vi "IMAQ-SaveVideo.vi"(1 "Exposure Time (ms)":u32, 2 "Image":T1, 3 "Grabar":refnum<vi>, 4 "Compression Filter":string) -> (0 "Selected Path for AVI":path)   [LabVIEW 2010]
uses:
  <vilib>/vision/Image Controls.llb/IMAQ Image.ctl
  <vilib>/vision/Avi1.llb/AviRefnum.ctl
  <vilib>/Utility/error.llb/DialogType.ctl
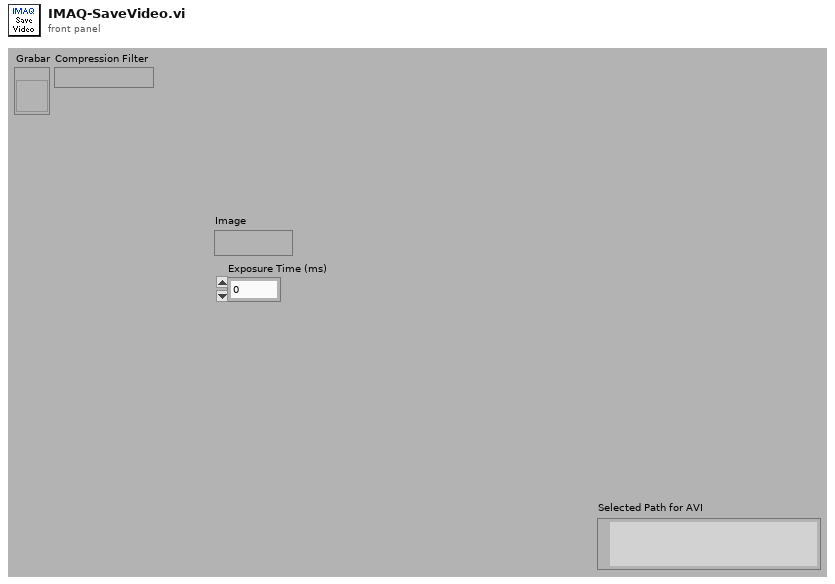
[diagram p1: front panel]
types:
  T1 = typedef "IMAQ Image.ctl" = refnum<image>
  T2 = typedef "AviRefnum.ctl" = refnum<k1>
  T3 = enum32{"existing file", "new file", "new or existing file", "existing dir", "new dir", "new or existing dir", "existing file (use LLBs)", "new file (use LLBs)", "new or existing file (use LLBs)", "new or existing file or directory (use LLBs)"}
  T4 = typedef "DialogType.ctl" = u16
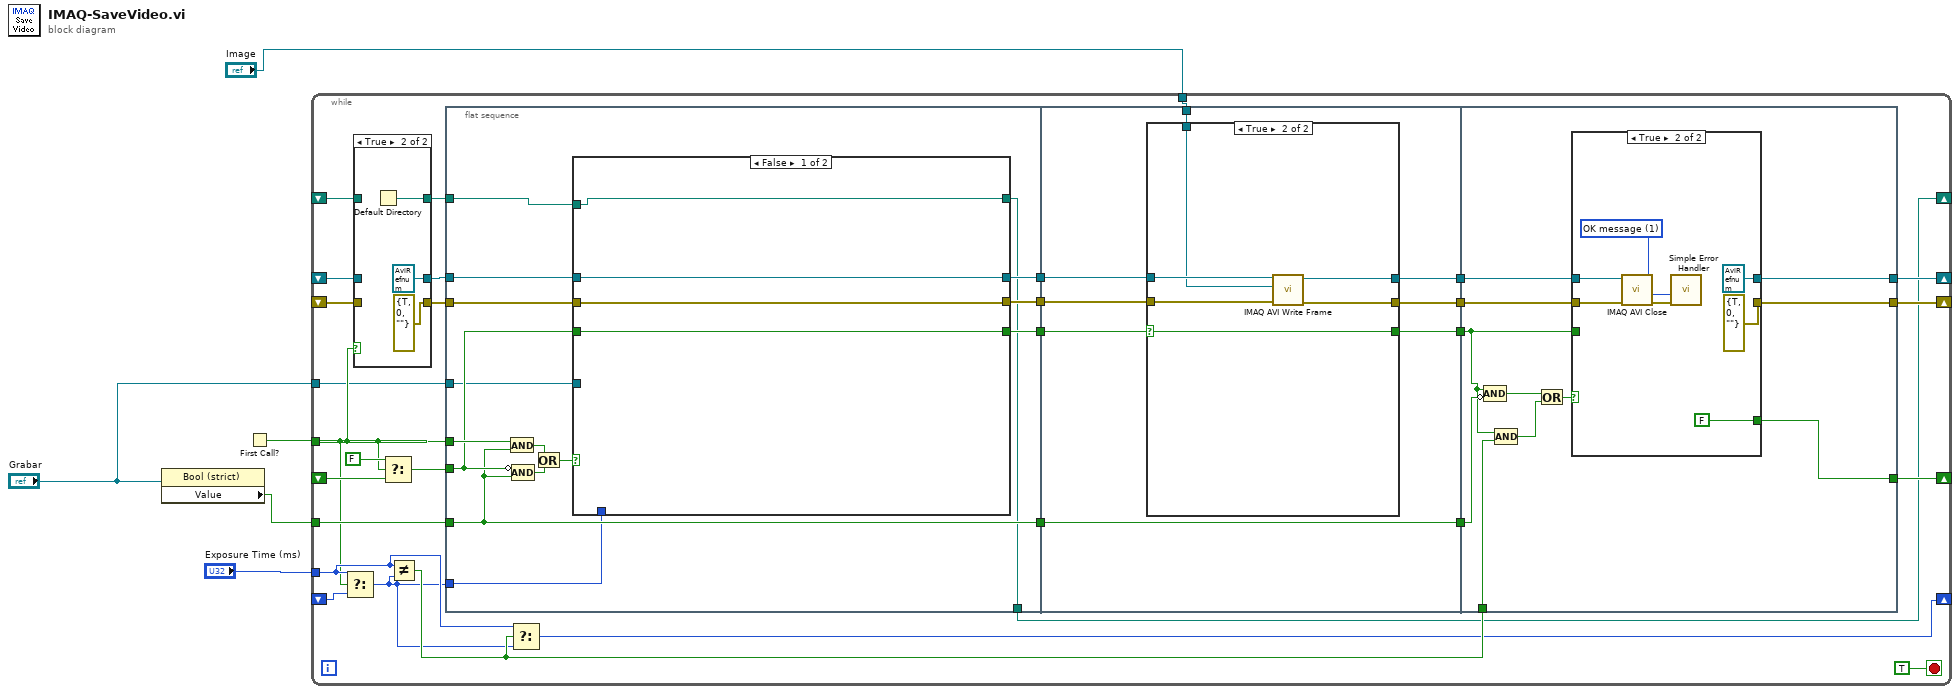
[diagram p0: block diagram]
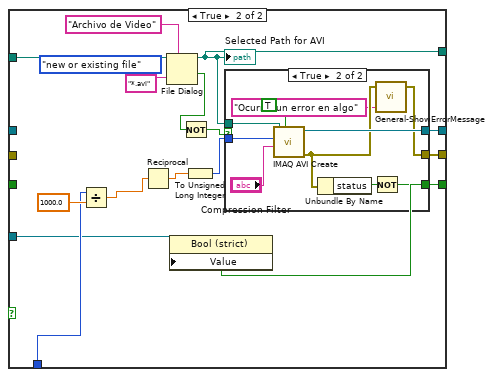
[diagram p3: hidden frame]
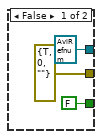
[diagram p4: hidden frame]
diagram:
  n1 = property class="Bool (strict)"(reference="Grabar") -> ("Value"=w2:bool)  [unwired: 1 in, 2 out]
  n2 = First Call?() -> (First Call?: T/F=w5:bool)
  n3 = while {
    tunnel: w5 -> [w10]
    tunnel: w2 -> [w35]
    shift-right: [w20] -> _
    shift-left: _ -> [w33]
    tunnel: "Image" -> [w29]
    shift-right: [w25] -> _
    shift-left: _ -> [w13]
    shift-right: [w24] -> _
    shift-left: _ -> [w11]
    tunnel: "Exposure Time (ms)" -> [w17]
    shift-right: [w15] -> _
    shift-left: _ -> [w19]
    tunnel: "Grabar" -> [w9]
    shift-right: [w7] -> _
    shift-left: _ -> [w8]
    stop <- TRUE stop-if-true
    n4 = Select(t=w17, s=w10, f=w19) -> (s? t:f=w16:u32)
    n5 = case shown="True" w10 {
      tunnel: [w39 T2 refnum ("Avi Refnum (duplicate)")] -> w14
      tunnel: w13 -> [w39 _]
      tunnel: [w38 errorcluster {"status"=TRUE, "code"=0, "source"=""} ("error out")] -> w12
      tunnel: w11 -> [w38 _]
      tunnel: w8 -> [w37 _]
      tunnel: [w37 w40] -> w6
      frame False {
      }
      frame True {
        n6 = Default Directory() -> (w40:path)
      }
    }
    n7 = Select(t=FALSE, s=w10, f=w33) -> (s? t:f=w32:bool)
    n8 = Not Equal?(x=w17, y=w16) -> (x != y?=w18:bool)
    n9 = flat-sequence {
      tunnel: w10 -> [w54]
      tunnel: w35 -> [w47]
      tunnel: w32 -> [w50]
      tunnel: [w53] -> w31
      tunnel: [w52] -> w30
      tunnel: [w51] -> w28
      tunnel: w14 -> [w49]
      tunnel: w12 -> [w48]
      tunnel: [w47] -> w23
      tunnel: w16 -> [w46]
      tunnel: w9 -> [w45]
      tunnel: w6 -> [w44]
      tunnel: [w43] -> w7
      tunnel: w31 -> [w97]
      tunnel: w30 -> [w96]
      tunnel: w29 -> [w95]
      tunnel: w28 -> [w94]
      tunnel: [w93] -> w27
      tunnel: [w92] -> w26
      tunnel: w23 -> [w91]
      tunnel: [w91] -> w22
      tunnel: [w90] -> w21
      tunnel: w27 -> [w117]
      tunnel: w26 -> [w116]
      tunnel: [w115] -> w25
      tunnel: [w114] -> w24
      tunnel: w22 -> [w113]
      tunnel: w21 -> [w108]
      tunnel: [w112] -> w20
      tunnel: w18 -> [w109]
      frame #0 {
        n10 = And(x=w54, y=w47) -> (x .and. y?=w56:bool)
        n11 = Compound Arithmetic op=AND(invert w50, w47) -> (w55:bool)
        n12 = Or(x=w56, y=w55) -> (x .or. y?=w57:bool)
        n13 = case shown="False" w57 {
          tunnel: [w59 w66] -> w53
          tunnel: [w60 w70] -> w52
          tunnel: [w61 w67] -> w51
          tunnel: w50 -> [w61 _]
          tunnel: w49 -> [w60 _]
          tunnel: w48 -> [w59 _]
          tunnel: w46 -> [_ w69]
          tunnel: w45 -> [_ w68]
          tunnel: [w58 w63] -> w43
          tunnel: w44 -> [w58 w62]
          frame False {
          }
          frame True {
            (unwired) T3."new or existing file" ("select mode (2)")
            n14 = Divide(x=w69, y=1000.0) -> (x/y=w73:dbl)
            n15 = Reciprocal(x=w73) -> (1/x=w72:dbl)
            n16 = File Dialog(6:"*.avi" ("pattern"), 7:"Archivo de Video" ("prompt"), 11:w62) -> (1:w64:bool, 3:w63:path)  [unwired: 1 in, 5 out]
            "Selected Path for AVI" <- w63
            n17 = Not(x=w64) -> (.not. x?=w65:bool)
            n18 = To Unsigned Long Integer(number=w72) -> (unsigned 32bit integer=w71:u32)
            n19 = case shown="True" w65 {
              tunnel: w63 -> [_ w89]
              tunnel: w71 -> [_ w87]
              tunnel: [T2 refnum ("Avi Refnum") w85] -> w70
              tunnel: [FALSE w84] -> w67
              tunnel: [errorcluster {"status"=TRUE, "code"=0, "source"=""} ("Error OUT") w82] -> w66
              frame False {
              }
              frame True {
                n20 = call "IMAQ AVI Create"("Has Data"=TRUE, "Compression Filter"="Compression Filter", "Frames Per Second"=w87, "AVI Path"=w89) -> ("error out"=w83:errorcluster, "Avi Refnum"=w85:T2)  [unwired: 6 in]
                n21 = Unbundle By Name(w83) -> ("status"=w86:bool)
                n22 = Not(x=w86) -> (.not. x?=w84:bool)
                n23 = call "General-ShowErrorMessage.vi"("message"="Ocurrio un error en algo", "Error IN"=w83) -> ("Error OUT"=w82:errorcluster)  [unwired: 3 in]
              }
            }
            n24 = property class="Bool (strict)"(reference=w68, "Value"=w67) -> ()  [unwired: 1 in, 2 out]
          }
        }
      }
      frame #1 {
        n25 = case shown="True" w94 {
          selector: w94 -> [w98 w101]
          tunnel: w97 -> [w99 w106]
          tunnel: w96 -> [w100 w105]
          tunnel: w95 -> [_ w104]
          tunnel: [w99 w103] -> w93
          tunnel: [w100 w102] -> w92
          tunnel: [w98 w101] -> w90
          frame False {
          }
          frame True {
            n26 = call "IMAQ AVI Write Frame"("error in (no error)"=w106, "Image"=w104, "Avi Refnum"=w105) -> ("error out"=w103:errorcluster, "Avi Refnum (duplicate)"=w102:T2)  [unwired: 1 in, 6 out]
          }
        }
      }
      frame #2 {
        n27 = Compound Arithmetic op=AND(w108, invert w113) -> (w111:bool)
        n28 = Compound Arithmetic op=AND(w108, w109) -> (w107:bool)
        n29 = Or(x=w111, y=w107) -> (x .or. y?=w110:bool)
        n30 = case shown="True" w110 {
          tunnel: w117 -> [w119 w125]
          tunnel: w116 -> [w120 w126]
          tunnel: [w120 T2 refnum ("Avi Refnum (duplicate)")] -> w115
          tunnel: [w119 errorcluster {"status"=TRUE, "code"=0, "source"=""} ("error out")] -> w114
          tunnel: [w118 FALSE] -> w112
          tunnel: w108 -> [w118 _]
          frame False {
          }
          frame True {
            w121 = T4 1 items=["no dialog", "OK message", "continue or stop message", "OK message + warnings", "continue/stop + warnings"] ("type of dialog (OK msg:1)")
            n31 = call "IMAQ AVI Close"("error in (no error)"=w125, "Avi Refnum"=w126) -> ("error out"=w127:errorcluster)  [unwired: 9 out]
            n32 = call <vilib>:"Simple Error Handler.vi"("type of dialog (OK msg:1)"=w121, "error in (no error)"=w127) -> ()  [unwired: 8 out]
          }
        }
      }
    }
    n33 = Select(t=w17, s=w18, f=w16) -> (s? t:f=w15:u32)
  }
